vi "HovaCAL fix Sollwerte in Tabelle.vi"(8 "error in (no error)":errorcluster caption="Fehler (Eingang, kein Fehler)", 11 "Anzahl Stufen":sgl) -> (0 "error out":errorcluster caption="Fehler (Ausgang)")   [LabVIEW 2020, in "Linearisierung v2.lvlib"]
uses:
  Linearisierung v2.lvlib
  Gasteiler/Aktionen FGV Gasteiler Daten.ctl
  GasteilerType.ctl
  Gasteiler/HovaCAL_Interface/Kommunikation/Aktion FGV HovaCAL Interface Autolin.ctl
  Aktion Lin Daten aufarbeiten.ctl
  Gasteiler/Gasteiler.lvlib
  Gasteiler/HovaCAL_Interface/Kommunikation/Kommunikation.lvlib
  Gasteiler/HovaCAL_Interface/Helper/Helper.lvlib
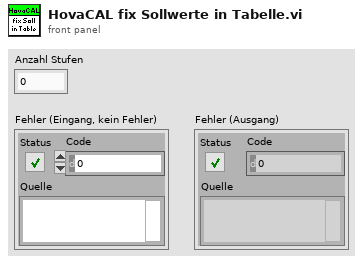
[diagram p1: front panel]
types:
  T1 = typedef "Linearisierung v2.lvlib/Gasteiler.lvlib/HovaCAL_Interface.lvlib/Kommunikation.lvlib/Aktion FGV HovaCAL Interface Autolin.ctl" = enum16{"lesen", "schreiben", "MFC Komponente fix setzen", "init"}
  T2 = typedef "Linearisierung v2.lvlib/GasteilerType.ctl" = u16
  T3 = typedef "Linearisierung v2.lvlib/Gasteiler.lvlib/Aktionen FGV Gasteiler Daten.ctl" = enum16{"lesen", "Gasteiler Daten", "Seriellen Param.", "MB-Endwert", "laden", "speichern", "Anforderung", "TCP", "Aufzeichnung Start"}
  T4 = typedef "Linearisierung v2.lvlib/Gasteiler.lvlib/Gasteiler Daten.ctl" = cluster{"Gasteiler":T5, "Gasteiler Stufen":T6, "Gasteiler Type":T2, "Konfig Gasteiler":T7, "Gasteiler Span Eingänge":u16}
  T5 = typedef "String - Eingabefeld.ctl" = string
  T6 = typedef "Linearisierung v2.lvlib/Gasteiler.lvlib/Gasteiler Stufen.ctl" = u16
  T7 = typedef "System Einstellungen V2.lvlib/Gasteiler Auswahl.ctl" = u16
  T8 = typedef "Linearisierung v2.lvlib/Aktion Lin Daten aufarbeiten.ctl" = enum16{"lesen", "Protkolldaten", "speichern", "laden", "EPA auswerten", "Tabelle schreiben", "Lin auswerten", "Tab init", "Stufentabelle", "EPA aktiviert", "Nachbehandlung laden", "Tabelle löschen", "Istwerte löschen", "Zeile löschen", "Zeile einfügen", "LIN aktiviert", "LIN/EPA aktiv laden", "EGAK Tab", "LIN übernehmen", "Tab init ohne Stufen"}
  T9 = typedef "Auswahlfeld.ctl" = u16
  T10 = typedef "Linearisierung v2.lvlib/Eingabetabelle.ctl" = string[][]
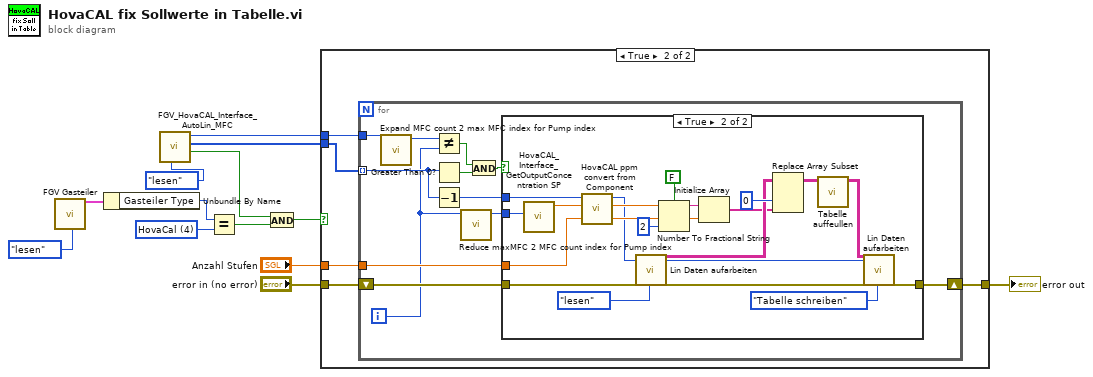
[diagram p0: block diagram]
diagram:
  w11 = T2 4 items=["LNI", "Analog-Display", "AVL GDU", "Horiba GDC", "HovaCal", "Horiba SGD 710C"] ("y")
  n1 = call "FGV Gasteiler.vi"("Aktionen"=Aktionen_FGV_Gasteiler_Daten."lesen") -> ("Gasteiler Daten"=w10:T4)  [unwired: 11 in, 7 out]
  n2 = Unbundle By Name(w10) -> ("Gasteiler Type"=w12:T2)
  n3 = call "FGV_HovaCAL_Interface_AutoLin_MFC.vi"("Aktion"=Aktion_FGV_HovaCAL_Interface_Autolin."lesen") -> ("fix conf"=w6:bool, "MFV Komponente fix out"=w5:u16[], "AutoLin MFC out"=w1:u16)  [unwired: 7 in, 1 out]
  n4 = Equal?(x=w12, y=w11) -> (x = y?=w9:bool)
  n5 = And(x=w6, y=w9) -> (x .and. y?=w7:bool)
  n6 = case shown="True" w7 {
    tunnel: w5 -> [_ w19]
    tunnel: "Anzahl Stufen" -> [_ w17]
    tunnel: "error in (no error)" -> [w14 w16]
    tunnel: [w14 w15] -> w2
    tunnel: w1 -> [_ w18]
    frame False {
    }
    frame True {
      n7 = for {
        tunnel: w19 -> [w30] mode=indexing
        tunnel: w17 -> [w29]
        shift-right: [w27] -> w15
        shift-left: w16 -> [w28]
        tunnel: w18 -> [w23]
        i -> [w21]
        n8 = call "Expand MFC count 2 max MFC index for Pump index.vi"("AutoLin MFC"=w23) -> ("MFC idx"=w22:i32)  [unwired: 8 in, 2 out]
        n9 = Not Equal?(x=w22, y=w21) -> (x != y?=w24:bool)
        n10 = Greater Than 0?(x=w30) -> (x > 0?=w31:bool)
        n11 = Decrement(x=w30) -> (x-1=w26:u16)
        n12 = call "Reduce maxMFC 2 MFC count index for Pump index.vi"("MFC idx"=w21) -> ("AutoLin MFC"=w20:i32)  [unwired: 8 in, 2 out]
        n13 = And(x=w24, y=w31) -> (x .and. y?=w25:bool)
        n14 = case shown="True" w25 {
          tunnel: w26 -> [_ w37]
          tunnel: w29 -> [_ w40]
          tunnel: w28 -> [w32 w39]
          tunnel: [w32 w38] -> w27
          tunnel: w20 -> [_ w35]
          frame False {
          }
          frame True {
            n15 = call "HovaCAL_Interface_GetOutputConcentration SP.vi"("AutoLin MFC Index"=w35) -> ("Konzentration"=w34:dbl)  [unwired: 8 in, 2 out]
            n16 = call "HovaCAL ppm convert from Component.vi"("Konzentration"=w34, "Gasnummer"=w37) -> ("Konzentration in %"=w36:dbl, "Gasnummer out"=w33:T9)  [unwired: 5 in, 3 out]
            n17 = call "Lin Daten aufarbeiten.vi"("Index (Seite)"=w33, "error in (no error)"=w39, "Aktionen"=Aktion_Lin_Daten_aufarbeiten."lesen") -> ("Eingabetabelle"=w48:T10, "Index (Seite) out"=w45:i32, "error out"=w46:errorcluster)  [unwired: 14 in, 8 out]
            n18 = Number To Fractional String(use system decimal point (T)=FALSE ("Systemdezimalzeichen verwenden (T)"), number=w36, precision (6)=i16 2 ("Genauigkeit (6)")) -> (F-format string=w43:string)  [unwired: 1 in]
            n19 = Initialize Array(w43, w40) -> (w44:string[])
            n20 = Replace Array Subset(array=w48, new element=w44, index (col)=0 ("Deaktivierter Index (Spalte)")) -> (w51:T10)  [unwired: 1 in]
            n21 = call "Tabelle auffeullen.vi"("Neue Tabelle"=w51) -> ("Tabelle"=w52:string[][])  [unwired: 10 in]
            n22 = call "Lin Daten aufarbeiten.vi"("Eingabetabelle"=w52, "Index (Seite)"=w45, "error in (no error)"=w46, "Aktionen"=Aktion_Lin_Daten_aufarbeiten."Tabelle schreiben") -> ("error out"=w38:errorcluster)  [unwired: 13 in, 10 out]
          }
        }
      }
    }
  }
  "error out" <- w2
